vi "Read U128 FIFO.vi"(2 "fifo":refnum<k21>, 12 "ready for output":bool=TRUE) -> (4 "output data":cluster{"high":u64, "low":u64}, 10 "output valid":bool)   [LabVIEW 2011, in "FIFO.lvlib"]
uses:
  <instrlib>/RF-RIO/FIFO/FIFO/FPGA/FIFO.lvlib
  <vilib>/rvi/DataTransferAndStorage/Container/Common/niFpgaContainerExecOnDevCompGetState.vi
  <vilib>/rvi/FIFO/Fifo_Resource/nirvififoEmulationSetSize.vi
  <vilib>/rvi/DataTransferAndStorage/Container/Common/niFpgaContainerGetUniqueNameForEmu.vi
  <vilib>/rvi/interface/RandomDataEmulation/nirviRandomDataFPGAFIFO.vi
  <vilib>/rvi/interface/RandomDataEmulation/niFpgaRandomDataHandleErrors.vi
  <vilib>/rvi/eio/common/nirviEmuReportErrorAndStop.vi
  <vilib>/rvi/DataTransferAndStorage/Container/XNode/niFpgaContainer.xnode
  <vilib>/rvi/FIFO/Fifo_Resource/niFpgaFifoEmulationRefIn.vi
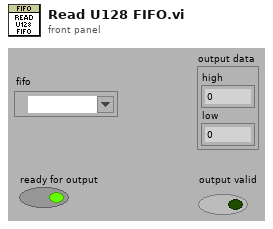
[diagram p1: front panel]
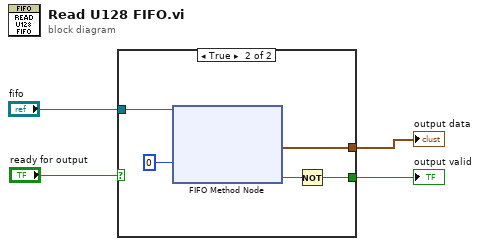
[diagram p0: block diagram]
diagram:
  n1 = case shown="True" "ready for output" {
    tunnel: [_ w5] -> w3
    tunnel: [_ w9] -> w2
    tunnel: "fifo" -> [_ w8]
    frame False {
    }
    frame True {
      n2 = xnode ("FIFO Method Node")("Timeout"=0, "FIFO In"=w8) -> ("Element"=w5:cluster{"high":u64, "low":u64}, "Timed Out?"=w6:bool)  [unwired: 1 out]
      n3 = Not(x=w6) -> (.not. x?=w9:bool)
    }
  }
  "output valid" <- w2
  "output data" <- w3
